vi "Voltech PM1000+ Integrator Measurement.vi"() -> ()   [LabVIEW 2015]
doc: "The purpose of this vi is to show the basic measurements that PM1000+ can make. The results are returned using the FRD command. This returns the results that are shown on the screen, in the order in which they appear on the screen. As results are selected using comms, the results are added to the bottom of the list, with the exception of harmonics, which always appear at the end of the list."
uses:
  <vilib>/Utility/error.llb/DialogType.ctl
  <instrlib>/Voltech PM1000+/Public/Configure/Configure Measurements (Integrator).vi
  <instrlib>/Voltech PM1000+/Voltech PM1000+.lvlib
panel:
  in  "Serial Configuration":T1={"Baud Rate"=19200, "Parity"=0, "Data Bits"=8, "Stop Bits"=10, "Flow Control"=2} {"Flow Control" items=["None"=0, "RTS/CTS"=2]; "Stop Bits" items=["1.0"=10]; "Data Bits" items=["8"=8]; "Parity" items=["None"]; "Baud Rate" items=["9600"=9600, "19200"=19200, "38400"=38400]}
  in  "Reset Integrator":bool
  in  "Stop Integrator":bool
  in  "Start Integrator":bool
  in  "Reset/Stop Integrator":bool=TRUE
  out "Number of Measurements Taken":u32
  out "error out":errorcluster
  in  "error in (no error)":errorcluster
  in  "Do ID Query":bool=TRUE
  in  "Do *RST":bool=TRUE
  in  "Select Mode (Normal)":u16(ring)=4 items=["Normal", "Ballast", "Inrush", "Standby Power", "Integrator"]
  in  "Enable Autozero  (True)":bool=TRUE caption="Autozero  (Enable)"
  in  "Enable Blanking (True)":bool=TRUE
  in  "Shunt (Internal)":u16(ring) items=["Internal", "External"]
  in  "Freq Source (Voltage)":u16(ring) items=["Voltage", "Current"]
  in  "Measurements":cluster{"Integrator Measurements":i32[]}={"Integrator Measurements"=[0, 1, 5, 6, 8]}
  in  "Fixed/Auto Ranging":T2 {"Volts Ranging (Auto)" items=["Auto", "10Vpk", "46Vpk", "215Vpk", "900Vpk"]; "Amps Ranging (Auto)" items=["Auto", "0.1Apk", "0.4Apk", "1.6Apk", "6.25Apk", "25Apk", "100Apk"]}
  in  "Scaling":T3={"Voltage Sacling (1.0000)"=1.0, "Current Sacling (1.0000)"=1.0} {"Current Sacling (1.0000)" min=1e-06 max=1000000.0 step=1.0 format="%.6f"; "Voltage Sacling (1.0000)" min=1e-06 max=1000000.0 step=1.0 format="%.6f"}
  in  "VISA resource name":refnum<visa-resource-name>
  in  "stop":bool
  out "Parameter":string[](array[string])
  out "Value":dbl[](array[numeric])
  # "(c) 2008-2009 Voltech Instruments.  ALL RIGHTS RESERVED."
  # "Configuration Side"
  # "1. Leave it as default or set up the PM1000+ instruments on the left  \n    \"Configuration Side\".\n2. Press Ctrl+R to run the test.\n3. Press the lower right side \"STOP\" button to stop the test."
  # "Loop Controls"
  # "Results Side"
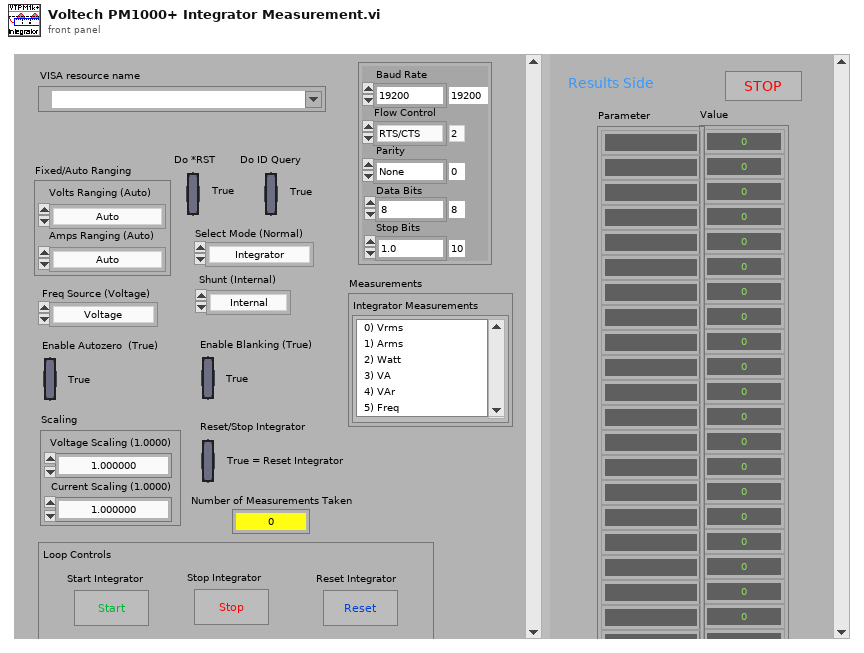
[diagram p1: front panel]
types:
  T1 = cluster{"Baud Rate":u32, "Parity":u16, "Data Bits":u16, "Stop Bits":u16, "Flow Control":u16}
  T2 = cluster{"Amps Ranging (Auto)":u16, "Volts Ranging (Auto)":u16}
  T3 = cluster{"Voltage Sacling (1.0000)":dbl, "Current Sacling (1.0000)":dbl}
  T4 = typedef "DialogType.ctl" = u16
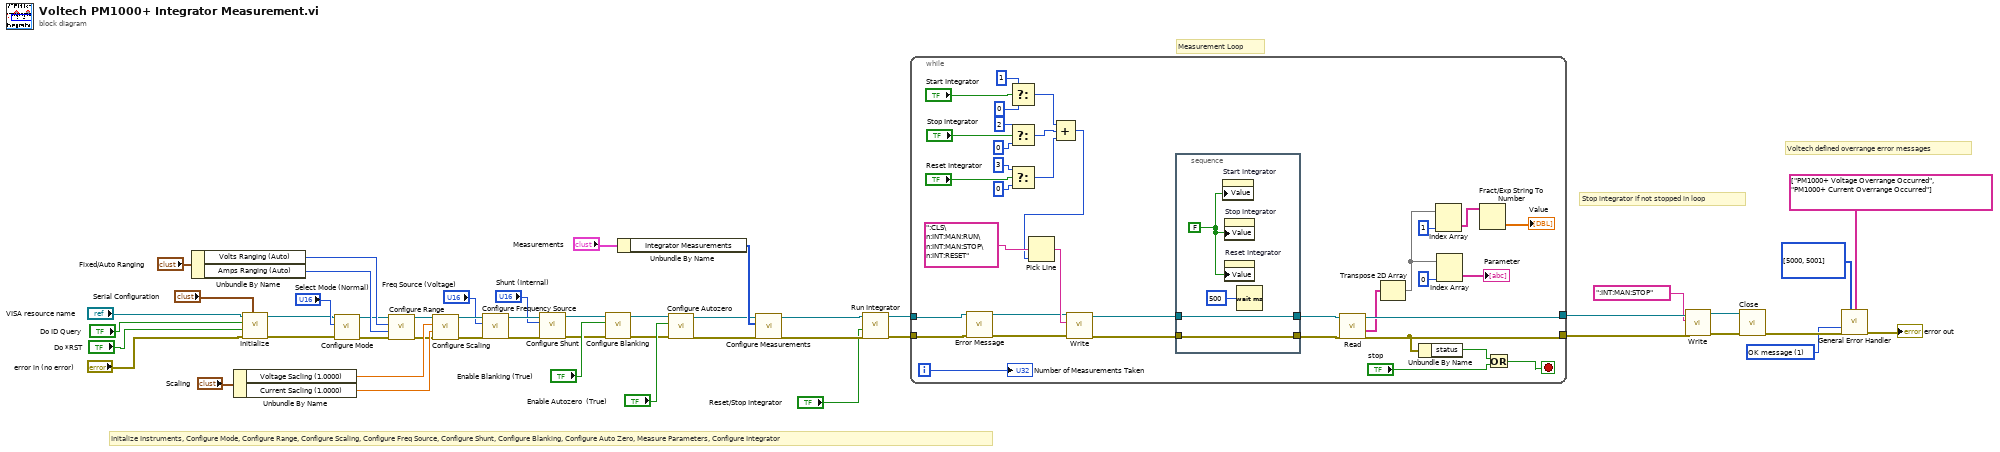
[diagram p0: block diagram]
diagram:
  w17 = T4 1 items=["no dialog", "OK message", "continue or stop message", "OK message + warnings", "continue/stop + warnings"] ("type of dialog (OK msg:1)")
  # "Voltech defined overrange error messages"
  # "Measurement Loop"
  # "Stop integrator if not stopped in loop"
  # "Initalize Instruments, Configure Mode, Configure Range, Configure Scaling, Configure Freq Source, Configure Shunt, Configure Blanking, Configure Auto Zero, Measure Parameters, Configure Integrator"
  n1 = Unbundle By Name("Fixed/Auto Ranging") -> ("Volts Ranging (Auto)"=w41:u16, "Amps Ranging (Auto)"=w40:u16)
  n2 = Unbundle By Name("Scaling") -> ("Voltage Sacling (1.0000)"=w44:dbl, "Current Sacling (1.0000)"=w43:dbl)
  n3 = call <instrlib>:"Initialize.vi"("Serial Configuration"="Serial Configuration", "error in (no error)"="error in (no error)", "Reset (True)"="Do *RST", "ID Query (True)"="Do ID Query", "VISA resource name"="VISA resource name") -> ("error out"=w5:errorcluster, "VISA resource name out"=w6:refnum<visa-resource-name>)  [unwired: 5 in]
  n4 = call <instrlib>:"Configure Mode.vi"("error in (no error)"=w5, "Select Mode (Normal)"="Select Mode (Normal)", "VISA resource name"=w6) -> ("error out"=w9:errorcluster, "VISA resource name out"=w10:refnum<visa-resource-name>)  [unwired: 7 in]
  n5 = call <instrlib>:"Configure Range.vi"("error in (no error)"=w9, "Current Range (Auto)"=w40, "Voltage Range (Auto)"=w41, "VISA resource name"=w10) -> ("error out"=w11:errorcluster, "VISA resource name out"=w12:refnum<visa-resource-name>)  [unwired: 6 in]
  n6 = call <instrlib>:"Configure Scaling.vi"("error in (no error)"=w11, "Current Sacling (1.0000)"=w43, "Voltage Sacling (1.0000)"=w44, "VISA resource name"=w12) -> ("error out"=w46:errorcluster, "VISA resource name out"=w47:refnum<visa-resource-name>)  [unwired: 6 in]
  n7 = call <instrlib>:"Configure Frequency Source.vi"("error in (no error)"=w46, "Frequency Source (Voltage)"="Freq Source (Voltage)", "VISA resource name"=w47) -> ("error out"=w49:errorcluster, "VISA resource name out"=w48:refnum<visa-resource-name>)  [unwired: 7 in]
  n8 = call <instrlib>:"Configure Shunt.vi"("error in (no error)"=w49, "Shunt (Internal)"="Shunt (Internal)", "VISA resource name"=w48) -> ("error out"=w34:errorcluster, "VISA resource name out"=w33:refnum<visa-resource-name>)  [unwired: 7 in]
  n9 = call <instrlib>:"Configure Blanking.vi"("error in (no error)"=w34, "Enable Blanking (True)"="Enable Blanking (True)", "VISA resource name"=w33) -> ("error out"=w31:errorcluster, "VISA resource name out"=w32:refnum<visa-resource-name>)  [unwired: 7 in]
  n10 = Unbundle By Name("Measurements") -> ("Integrator Measurements"=w30:i32[])
  n11 = call <instrlib>:"Configure Autozero.vi"("error in (no error)"=w31, "Enable Autozero (True)"="Enable Autozero  (True)", "VISA resource name"=w32) -> ("error out"=w13:errorcluster, "VISA resource name out"=w14:refnum<visa-resource-name>)  [unwired: 7 in]
  n12 = call-poly <instrlib>:"Configure Measurements.vi"("error in (no error)"=w13, "Integrator Measurements"=w30, "VISA resource name"=w14) -> ("error out"=w28:errorcluster, "VISA resource name out"=w29:refnum<visa-resource-name>)  [unwired: 7 in]
  n13 = call <instrlib>:"Run Integrator.vi"("error in (no error)"=w28, "Reset/Stop Integrator (False)"="Reset/Stop Integrator", "VISA resource name"=w29) -> ("error out"=w26:errorcluster, "VISA resource name out"=w25:refnum<visa-resource-name>)  [unwired: 7 in]
  n14 = while {
    tunnel: w25 -> [w55]
    tunnel: w26 -> [w54]
    tunnel: [w83] -> w24
    tunnel: [w53] -> w23
    i -> [w85]
    stop <- w50 stop-if-true
    n15 = call <instrlib>:"Error Message.vi"("VISA resource name"=w55, "error in (no error)"=w54) -> ("VISA resource name out"=w57:refnum<visa-resource-name>, "error out"=w56:errorcluster)  [unwired: 12 in]
    n16 = Select(t=1, s="Start Integrator", f=0) -> (s? t:f=w65:i32)
    n17 = Select(t=2, s="Stop Integrator", f=0) -> (s? t:f=w64:i32)
    n18 = Select(t=3, s="Reset Integrator", f=0) -> (s? t:f=w63:i32)
    n19 = Compound Arithmetic op=ADD(w65, w64, w63) -> (w62:i32)
    n20 = Pick Line(multi-line string=":CLS\n:INT:MAN:RUN\n:INT:MAN:STOP\n:INT:RESET", line index=w62) -> (output string=w82:string)  [unwired: 1 in]
    n21 = call <instrlib>:"Write.vi"("error in (no error)"=w56, "Write Buffer"=w82, "VISA resource name"=w57) -> ("error out"=w59:errorcluster, "VISA resource name out"=w61:refnum<visa-resource-name>)  [unwired: 7 in]
    n22 = stacked-sequence {
      tunnel: [w88] -> w60
      tunnel: w61 -> [w88]
      tunnel: w59 -> [w87]
      tunnel: [w87] -> w58
      frame #0 {
        w89 = FALSE
        n23 = property on="Start Integrator" class="Bool (strict)"("Value"=w89) -> ()  [unwired: 2 in, 2 out]
        n24 = property on="Stop Integrator" class="Bool (strict)"("Value"=w89) -> ()  [unwired: 2 in, 2 out]
        n25 = property on="Reset Integrator" class="Bool (strict)"("Value"=w89) -> ()  [unwired: 2 in, 2 out]
        n26 = Wait (ms)(milliseconds to wait=500) -> ()  [unwired: 1 out]
      }
    }
    n27 = call <instrlib>:"Read.vi"("error in (no error)"=w58, "VISA resource name"=w60) -> ("error out"=w53:errorcluster, "Measurement Results"=w81:string[][], "VISA resource name out"=w83:refnum<visa-resource-name>)  [unwired: 7 in]
    n28 = Transpose 2D Array(2D array=w81) -> (transposed array=w80:string[][])
    n29 = Unbundle By Name(w53) -> ("status"=w52:bool)
    n30 = Index Array(array=w80, index (col)=1) -> (element=w77:string[])  [unwired: 1 in]
    n31 = Index Array(array=w80, index (col)=0) -> (element=→"Parameter":string[])  [unwired: 1 in]
    n32 = Fract/Exp String To Number(string=w77) -> (number=→"Value":dbl[])  [unwired: 3 in, 1 out]
    n33 = Or(x=w52, y="stop") -> (x .or. y?=w50:bool)
    "Number of Measurements Taken" <- w85
  }
  n34 = call <instrlib>:"Write.vi"("error in (no error)"=w23, "Write Buffer"=":INT:MAN:STOP", "VISA resource name"=w24) -> ("error out"=w21:errorcluster, "VISA resource name out"=w22:refnum<visa-resource-name>)  [unwired: 7 in]
  n35 = call <instrlib>:"Close.vi"("error in (no error)"=w21, "VISA resource name"=w22) -> ("error out"=w18:errorcluster)  [unwired: 9 in]
  n36 = call <vilib>:"General Error Handler.vi"("[user-defined codes]"=i32[] [5000, 5001], "[user-defined descriptions]"=string[] ["PM1000+ Voltage Overrange Occurred", "PM1000+ Current Overrange Occurred"], "type of dialog (OK msg:1)"=w17, "error in (no error)"=w18) -> ("error out"=→"error out":errorcluster)  [unwired: 7 in, 4 out]
